vi "Write Sessions.vi"(10 "Sessions":refnum<class "Session.lvclass">[](array[class]), 11 "TCPConnectionHandler in":refnum<class "TCPConnectionHandler.lvclass">) -> (3 "TCPConnectionHandler out":refnum<class "TCPConnectionHandler.lvclass">)   [LabVIEW 2013, in "MQTT Server.lvlib" / "TCPConnectionHandler.lvclass"]
uses:
  TCPConnectionHandler.lvclass
  Session/Session.lvclass
  TCPConnectionHandler.lvclass/TCPConnectionHandler.ctl
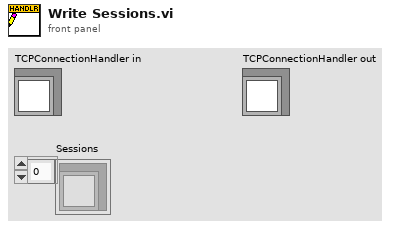
[diagram p1: front panel]
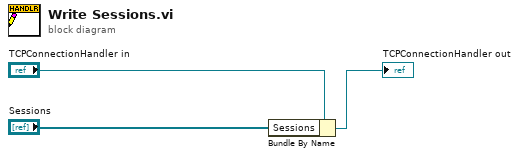
[diagram p0: block diagram]
diagram:
  n1 = Bundle By Name(cluster="TCPConnectionHandler in", "Sessions"="Sessions") -> (→"TCPConnectionHandler out":refnum<class "TCPConnectionHandler.lvclass">)
